vi "LEP_RV_MemoryMap_Query.vi"(8 "error in (no error)":errorcluster, 11 "Source File":path) -> (0 "error out":errorcluster, 3 "VI Config":T1)   [LabVIEW 2011]
doc: "Query the memory mapper database for memory section the passed c file should be placed in."
uses:
  <vilib>/LabVIEW Targets/Embedded/Utilities/MemMap/EMB_Utility_MemMap_VI_Config.ctl
  <vilib>/LabVIEW Targets/Embedded/Utilities/MemMap/EMB_Utility_MemMap_VI_Type.ctl
  <vilib>/Platform/EmbProject/Plugins/utilities/LEP_Utilities_GetSetProjectData_Variant.vi
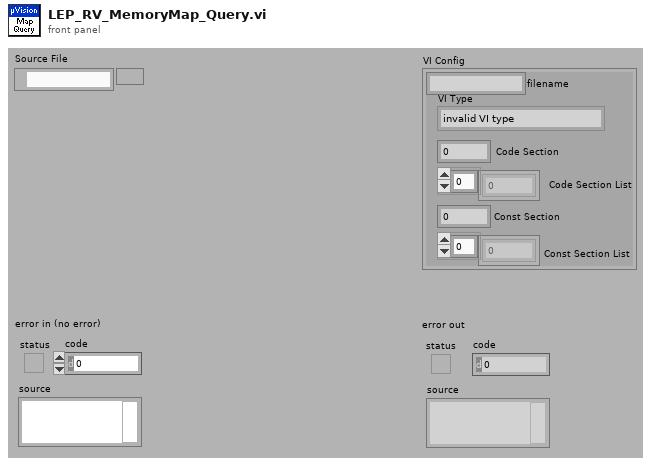
[diagram p1: front panel]
types:
  T1 = typedef "EMB_Utility_MemMap_VI_Config.ctl" = cluster{"filename":string, "Code Section":i32, "Code Section List":i32[], "Const Section":i32, "Const Section List":i32[], "VI Type":T2}
  T2 = typedef "EMB_Utility_MemMap_VI_Type.ctl" = enum32{"invalid VI type", "Standard VI", "Control VI", "Global VI", "Polymorphic VI", "Configuration VI", "SubSystem"}
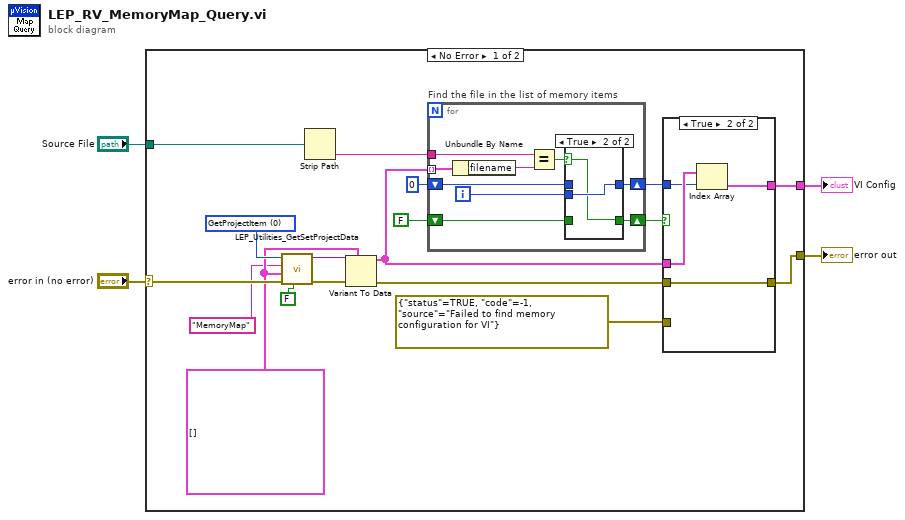
[diagram p0: block diagram]
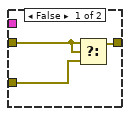
[diagram p2: hidden frame]
diagram:
  n1 = case shown="No Error" "error in (no error)" {
    selector: "error in (no error)" -> [w22 w43]
    tunnel: "Source File" -> [w13 _]
    tunnel: [w15 w43] -> w2
    tunnel: [w21 _] -> w3
    frame No Error {
      w7 = T1[] []
      w11 = u16 0 items=["GetProjectItem", "SetProjectItem"] ("Command")
      n2 = call-poly <vilib>:"LEP_Utilities_GetSetProjectData.vi"("access target data (F)"=FALSE ("Prefix target name?"), "error in"=w22, "Variant In"=w7, "ItemName"="MemoryMap", "Command"=w11) -> ("error out"=w9:errorcluster, "Variant Out"=w8:variant)  [unwired: 4 in, 1 out]
      n3 = Strip Path(path=w13) -> (name=w12:string)  [unwired: 1 out]
      n4 = Variant To Data(error in=w9, type=w7, Variant=w8) -> (data=w20:T1[], error out=w5:errorcluster)
      n5 = for "Find the file in the list of memory items" {
        tunnel: w20 -> [w38] mode=indexing
        shift-right: [w34] -> w18
        shift-left: 0 -> [w33]
        shift-right: [w32] -> w16
        shift-left: FALSE -> [w31]
        tunnel: w12 -> [w30]
        i -> [w35]
        n6 = Unbundle By Name(w38) -> ("filename"=w37:string)
        n7 = Equal?(x=w30, y=w37) -> (x = y?=w36:bool)
        n8 = case shown="True" w36 {
          selector: w36 -> [_ w41]
          tunnel: w35 -> [_ w42]
          tunnel: [w40 w42] -> w34
          tunnel: w33 -> [w40 _]
          tunnel: [w39 w41] -> w32
          tunnel: w31 -> [w39 _]
          frame False {
          }
          frame True {
          }
        }
      }
      n9 = case shown="True" w16 {
        tunnel: [_ w29] -> w21
        tunnel: w20 -> [_ w28]
        tunnel: w18 -> [_ w27]
        tunnel: [w24 w26] -> w15
        tunnel: w5 -> [w25 w26]
        tunnel: errorcluster {"status"=TRUE, "code"=-1, "source"="Failed to find memory configuration for VI"} ("f") -> [w23 _]
        frame False {
          n10 = Select(t=w25, s=w25, f=w23) -> (s? t:f=w24:errorcluster)
        }
        frame True {
          n11 = Index Array(array=w28, index=w27) -> (element=w29:T1)
        }
      }
    }
    frame Error {
    }
  }
  "VI Config" <- w3
  "error out" <- w2
